vi "group Bulk Write.vi"(10 "protocol_version":i32, 11 "port_num":i32) -> (3 "function return":i32)   [LabVIEW 2016, in "dxl_x86_c.lvlib"]
doc: "WINDECLSPEC int groupBulkWrite (int port_num, int protocol_version);"
uses:
  dxl_x86_c.lvlib
  dxl_x86_c.dll
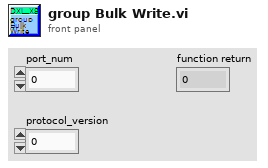
[diagram p1: front panel]
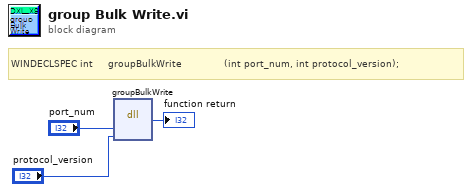
[diagram p0: block diagram]
diagram:
  # "WINDECLSPEC int     groupBulkWrite              (int port_num, int protocol_version);"
  n1 = dll-call lib="C:/Users/Platform/Desktop/DynamixelSDK/labview/dxl_x86_c.lvlib/dxl_x86_c.*" fn="groupBulkWrite"("port_num"="port_num", "protocol_version"="protocol_version") -> (→"function return":i32)  [unwired: 5 in, 2 out]
